vi "Search Unique Complex Numbers.vi"(8 "tolerance":dbl, 11 "Sorted numbers":cdb[](array[numeric]) format="%.2f") -> (3 "Unique numbers":cdb[](array[numeric]))   [LabVIEW 2017, in "NI_AALPro.lvlib"]
uses:
  <vilib>/Analysis/NI_AALPro.lvlib
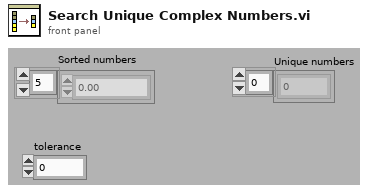
[diagram p1: front panel]
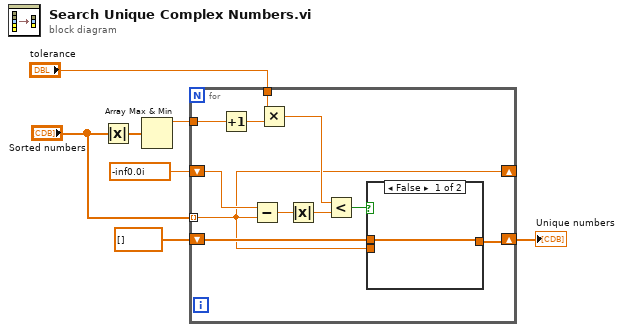
[diagram p0: block diagram]
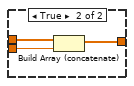
[diagram p2: hidden frame]
diagram:
  n1 = Absolute Value(x="Sorted numbers") -> (abs(x)=w5:dbl[])
  n2 = Array Max & Min(array=w5) -> (max value=w4:dbl)  [unwired: 3 out]
  n3 = for {
    shift-right: [w8] -> _
    shift-left: cdb -inf+0.0i -> [w9]
    tunnel: "Sorted numbers" -> [w8] mode=indexing
    shift-right: [w17] -> w1
    shift-left: cdb[] [] -> [w18]
    tunnel: w4 -> [w16]
    tunnel: "tolerance" -> [w15]
    n4 = Increment(x=w16) -> (x+1=w14:dbl)
    n5 = Subtract(x=w9, y=w8) -> (x-y=w11:cdb)
    n6 = Multiply(x=w15, y=w14) -> (x*y=w13:dbl)
    n7 = Absolute Value(x=w11) -> (abs(x)=w10:dbl)
    n8 = Less?(x=w13, y=w10) -> (x < y?=w12:bool)
    n9 = case shown="False" w12 {
      tunnel: w18 -> [w19 w22]
      tunnel: [w19 w21] -> w17
      tunnel: w8 -> [_ w20]
      frame False {
      }
      frame True {
        n10 = Build Array (concatenate)(w22, w20) -> (w21:cdb[])
      }
    }
  }
  "Unique numbers" <- w1
